vi "testSame.vi"(8 "error in (no error)":errorcluster) -> (0 "error out":errorcluster)   [LabVIEW 2019, in "AssertionTest.lvlib" / "AssertEquals.lvlib"]
uses:
  AssertEquals.lvlib
  Assertion/Assertion.lvlib
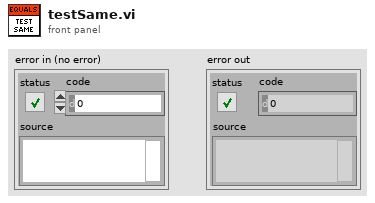
[diagram p1: front panel]
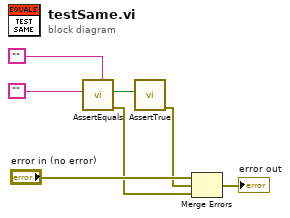
[diagram p0: block diagram]
diagram:
  n1 = call "AssertEquals.vi"("Expected"="", "Actual"="") -> ("error out"=w1:errorcluster, "Result"=w7:bool)  [unwired: 8 in]
  n2 = call "AssertTrue.vi"("Condition"=w7) -> ("error out"=w4:errorcluster)  [unwired: 9 in, 1 out]
  n3 = Merge Errors("error in (no error)", w4, w1) -> (→"error out":errorcluster)
